vi "Merged_Signals_2_Devices.vi"() -> ()   [LabVIEW 2017, in "Examples.lvlib"]
uses:
  Examples.lvlib
panel:
  out "Waveform Chart":dynamicdata(graph)
  in  "?":bool
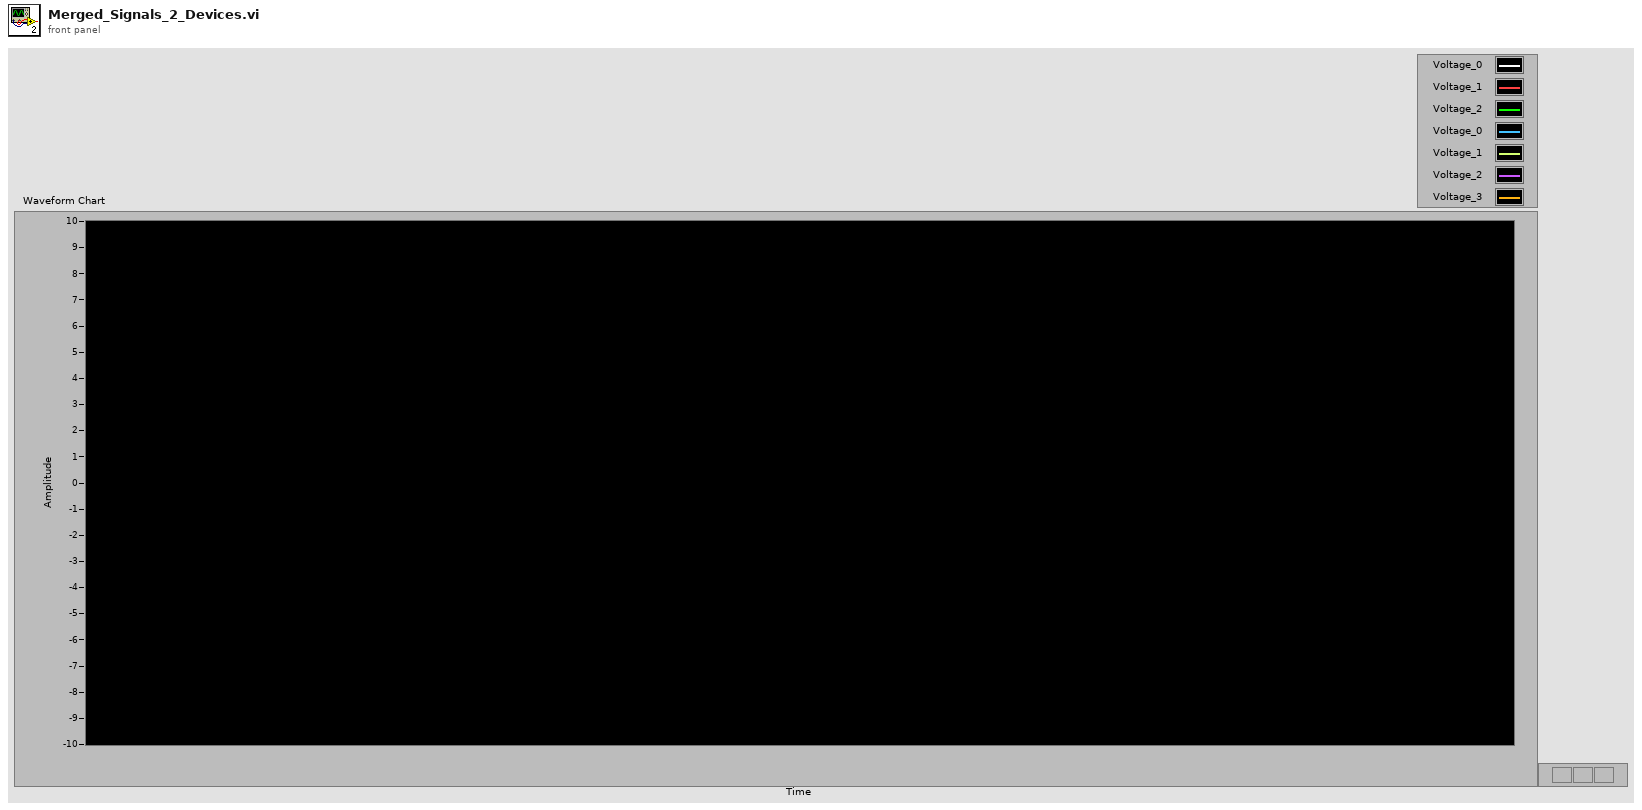
[diagram p1: front panel]
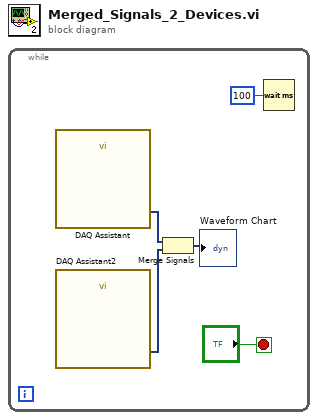
[diagram p0: block diagram]
diagram:
  n1 = while {
    stop <- "?" stop-if-true
    n2 = call "DAQ Assistant"() -> ("data"=w3:dynamicdata)  [unwired: 17 in, 2 out]
    n3 = call "DAQ Assistant2"() -> ("data"=w2:dynamicdata)  [unwired: 17 in, 2 out]
    n4 = Merge Signals(w3, w2) -> (→"Waveform Chart":dynamicdata)
    n5 = Wait (ms)(milliseconds to wait=u32 100) -> ()  [unwired: 1 out]
  }
